vi "lectura velocidad motores.vi"(6 "Periodo de muestreo [ s ]":dbl, 7 "read buffer":string, 9 "Resolucion encoder\n            Motor 3":dbl, 10 "Resolucion encoder\n            Motor 2":dbl, 11 "Resolucion encoder\n            Motor 1":dbl) -> (0 "Indicador de motor 3":bool, 1 "Velocidad motor 3":dbl[](array[numeric]), 2 "Indicador de motor  2":bool, 3 "Velocidad motor 2":dbl[](array[numeric]), 4 "Indicador de motor 1":bool, 5 "Velocidad motor 1":dbl[](array[numeric]))   [LabVIEW 2018]
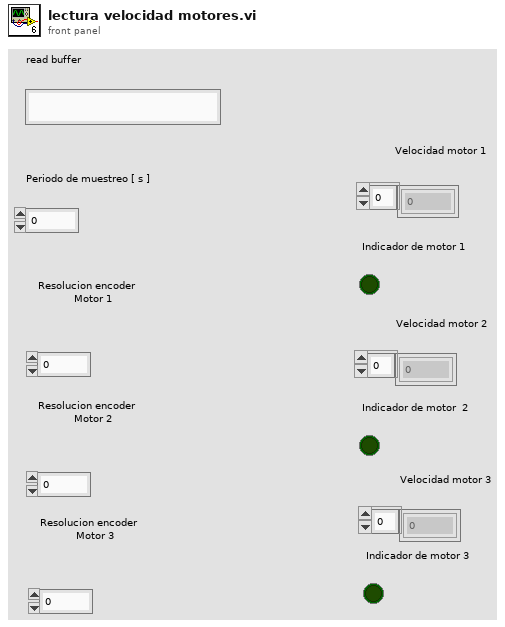
[diagram p1: front panel]
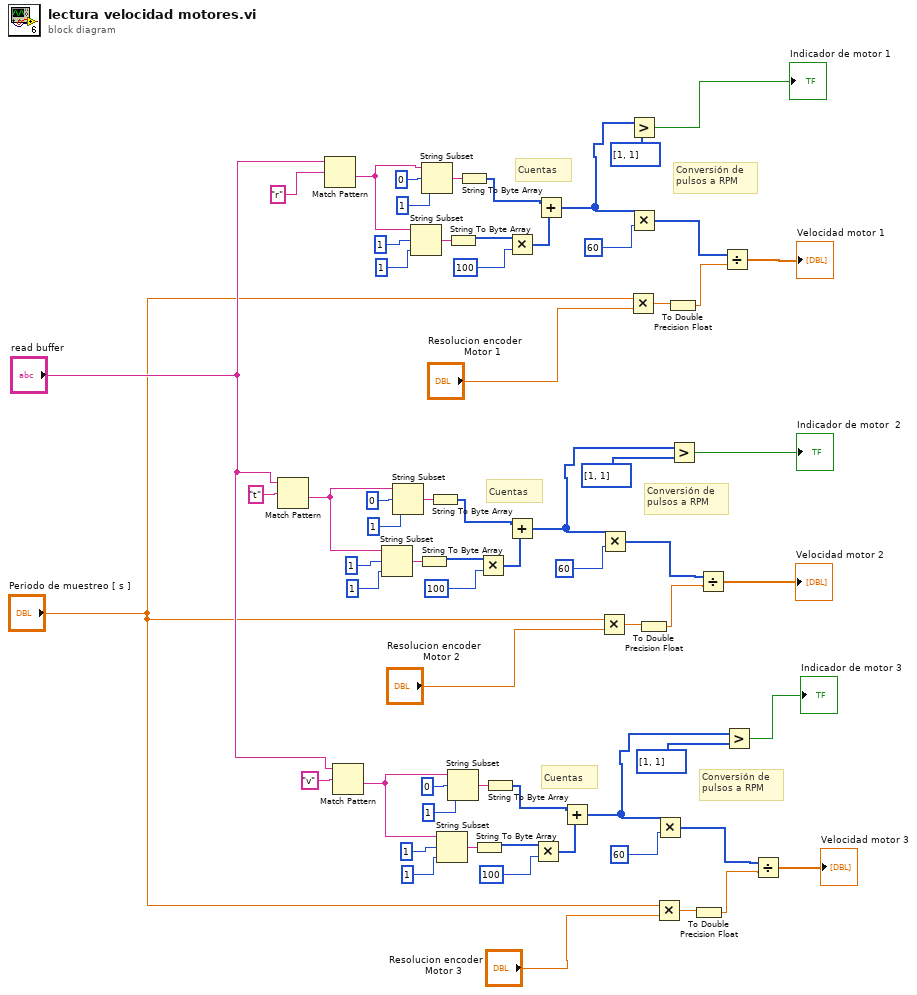
[diagram p0: block diagram]
diagram:
  # "Conversión de pulsos a RPM"
  # "Cuentas"
  # "Conversión de pulsos a RPM"
  # "Cuentas"
  # "Conversión de pulsos a RPM"
  # "Cuentas"
  n1 = Match Pattern(string="read buffer", regular expression="t") -> (after substring=w34:string)  [unwired: 1 in, 3 out]
  n2 = Match Pattern(string="read buffer", regular expression="r") -> (after substring=w35:string)  [unwired: 1 in, 3 out]
  n3 = Match Pattern(string="read buffer", regular expression="v") -> (after substring=w54:string)  [unwired: 1 in, 3 out]
  n4 = String Subset(string=w34, offset (0)=1, length (rest)=1 ("length (rest)")) -> (substring=w24:string)
  n5 = String Subset(string=w34, offset (0)=0, length (rest)=1 ("length (rest)")) -> (substring=w23:string)
  n6 = String Subset(string=w35, offset (0)=1, length (rest)=1 ("length (rest)")) -> (substring=w5:string)
  n7 = String To Byte Array(string=w24) -> (unsigned byte array=w27:u8[])
  n8 = String Subset(string=w35, offset (0)=0, length (rest)=1 ("length (rest)")) -> (substring=w4:string)
  n9 = String To Byte Array(string=w23) -> (unsigned byte array=w30:u8[])
  n10 = String Subset(string=w54, offset (0)=1, length (rest)=1 ("length (rest)")) -> (substring=w44:string)
  n11 = String To Byte Array(string=w5) -> (unsigned byte array=w8:u8[])
  n12 = String Subset(string=w54, offset (0)=0, length (rest)=1 ("length (rest)")) -> (substring=w43:string)
  n13 = String To Byte Array(string=w4) -> (unsigned byte array=w11:u8[])
  n14 = String To Byte Array(string=w44) -> (unsigned byte array=w47:u8[])
  n15 = Multiply(x=w27, y=100) -> (x*y=w29:i32[])
  n16 = String To Byte Array(string=w43) -> (unsigned byte array=w50:u8[])
  n17 = Multiply(x=w8, y=100) -> (x*y=w10:i32[])
  n18 = Add(x=w30, y=w29) -> (x+y=w36:i32[])
  n19 = Multiply(x=w47, y=100) -> (x*y=w49:i32[])
  n20 = Add(x=w11, y=w10) -> (x+y=w17:i32[])
  n21 = Add(x=w50, y=w49) -> (x+y=w55:i32[])
  n22 = Multiply(x="Periodo de muestreo [ s ]", y="Resolucion encoder\n            Motor 2") -> (x*y=w37:dbl)
  n23 = Multiply(x=w36, y=60) -> (x*y=w39:i32[])
  n24 = Multiply(x="Periodo de muestreo [ s ]", y="Resolucion encoder\n            Motor 1") -> (x*y=w16:dbl)
  n25 = Greater?(x=w17, y=i32[] [1, 1]) -> (0:→"Indicador de motor 1":bool)
  n26 = Multiply(x=w17, y=60) -> (x*y=w13:i32[])
  n27 = To Double Precision Float(number=w37) -> (double precision float=w40:dbl)
  n28 = Multiply(x="Periodo de muestreo [ s ]", y="Resolucion encoder\n            Motor 3") -> (x*y=w56:dbl)
  n29 = Multiply(x=w55, y=60) -> (x*y=w57:i32[])
  n30 = To Double Precision Float(number=w16) -> (double precision float=w14:dbl)
  n31 = Greater?(x=w36, y=i32[] [1, 1]) -> (0:→"Indicador de motor  2":bool)
  n32 = To Double Precision Float(number=w56) -> (double precision float=w58:dbl)
  n33 = Divide(x=w39, y=w40) -> (x/y=→"Velocidad motor 2":dbl[])
  n34 = Divide(x=w13, y=w14) -> (x/y=→"Velocidad motor 1":dbl[])
  n35 = Greater?(x=w55, y=i32[] [1, 1]) -> (0:→"Indicador de motor 3":bool)
  n36 = Divide(x=w57, y=w58) -> (x/y=→"Velocidad motor 3":dbl[])
